vi "Test tools list.vi"(8 "error in (no error)":errorcluster) -> (0 "error out":errorcluster, 3 "body":string)   [LabVIEW 2020, in "MCP Server tests.lvlib"]
uses:
  MCP Server tests.lvlib
  <vilib>/JDP Science/JSONtext/Next JSON Value.vi
  <vilib>/JDP Science/JSONtext/String Subset.vi
  <vilib>/JDP Science/JSONtext/Parsing/Advance past next JSON Value (inlined COPY).vi
  <vilib>/JDP Science/JSONtext/Parsing/Advance past whitespace.vi
  <vilib>/JDP Science/JSONtext/Parsing/Advance past String.vi
  <vilib>/JDP Science/JSONtext/Parsing/Advance past Number.vi
  <vilib>/JDP Science/JSONtext/Parsing/Advance past Line Ending.vi
  <vilib>/JDP Science/JSONtext/Parsing/Parse Full Path or Item Name.vi
  <vilib>/JDP Science/JSONtext/Parsing/Advance past Array.vi
  <vilib>/JDP Science/JSONtext/Parsing/Advance past Object.vi
  <vilib>/JDP Science/JSONtext/support/Error Cluster From Code.vi
  <vilib>/JDP Science/JSONtext/Offset/Find Item Locations by Path.vi
  <vilib>/addons/_JKI Toolkits/Caraya/classes/Test/Test.lvclass
  <vilib>/addons/_JKI Toolkits/Caraya/classes/Assert/Assert.lvclass
  <vilib>/JDP Science/JSONtext/JSONtext.lvlib
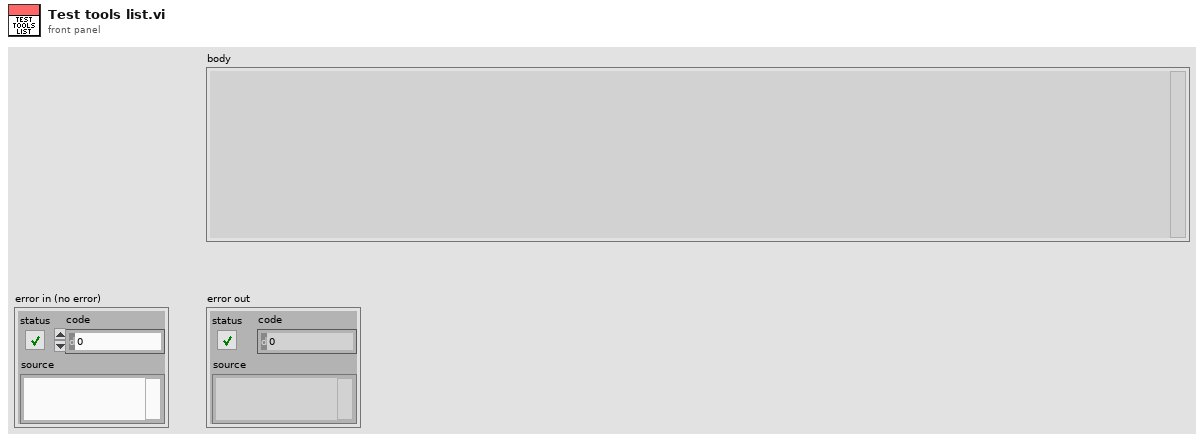
[diagram p1: front panel]
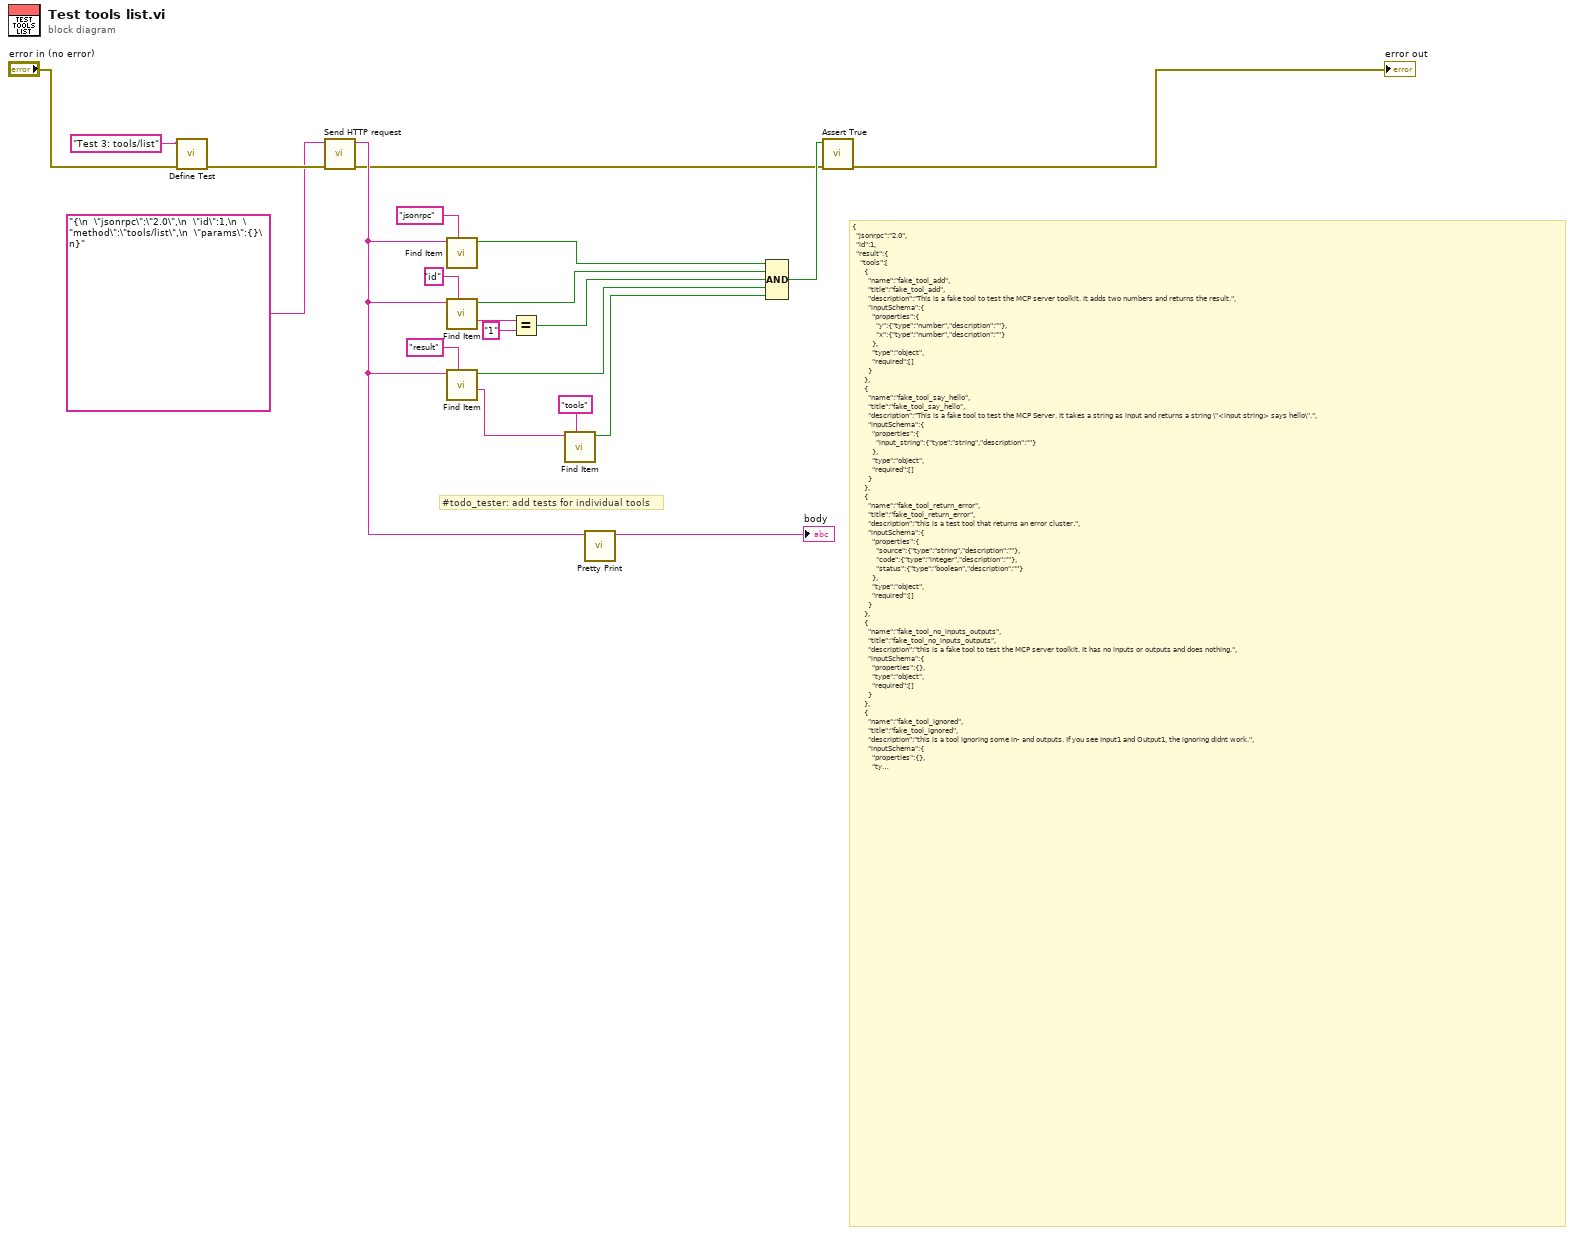
[diagram p0: block diagram]
diagram:
  # "#todo_tester: add tests for individual tools"
  # "{\n  \"jsonrpc\":\"2.0\",\n  \"id\":1,\n  \"result\":{\n    \"tools\":[\n      {\n        \"name\":\"fake_tool_add\",\n        \"title\":\"fake_tool_add\",\n        \"description\":\"This is a fake tool to test the MCP server toolkit. It adds two numbers and returns the result.\",\n        \"inputSchema\":{\n          \"properties\":{\n            \"y\":{\"type\":\"number\",\"description\":\"\"},\n            \"x\":{\"type\":\"number\",\"description\":\"\"}\n          },\n          \"type\":\"object\",\n          \"required\":[]\n        }\n      },\n      {\n        \"name\":\"fake_tool_say_hello\",\n        \"title\":\"fake_tool_say_hello\",\n        \"description\":\"This is a fake tool to test the MCP Server. It takes a string as input and returns a string \\\"<input string> says hello\\\".\",\n        \"inputSchema\":{\n          \"properties\":{\n            \"input_string\":{\"type\":\"string\",\"description\":\"\"}\n          },\n          \"type\":\"object\",\n          \"required\":[]\n        }\n      },\n      {\n        \"name\":\"fake_tool_return_error\",\n        \"title\":\"fake_tool_return_error\",\n        \"description\":\"this is a test tool that returns an error cluster.\",\n        \"inputSchema\":{\n          \"properties\":{\n            \"source\":{\"type\":\"string\",\"description\":\"\"},\n            \"code\":{\"type\":\"integer\",\"description\":\"\"},\n            \"status\":{\"type\":\"boolean\",\"description\":\"\"}\n          },\n          \"type\":\"object\",\n          \"required\":[]\n        }\n      },\n      {\n        \"name\":\"fake_tool_no_inputs_outputs\",\n        \"title\":\"fake_tool_no_inputs_outputs\",\n        \"description\":\"this is a fake tool to test the MCP server toolkit. It has no inputs or outputs and does nothing.\",\n        \"inputSchema\":{\n          \"properties\":{},\n          \"type\":\"object\",\n          \"required\":[]\n        }\n      },\n      {\n        \"name\":\"fake_tool_ignored\",\n        \"title\":\"fake_tool_ignored\",\n        \"description\":\"this is a tool ignoring some in- and outputs. If you see Input1 and Output1, the ignoring didnt work.\",\n        \"inputSchema\":{\n          \"properties\":{},\n          \"type\":\"object\",\n          \"required\":[]\n        }\n      }\n    ]\n  }\n}"
  n1 = call <vilib>:"Define Test.vi"("error in (no error)"="error in (no error)", "Label (VI Title)"="Test 3: tools/list") -> ("error out"=w8:errorcluster)  [unwired: 8 in, 1 out]
  n2 = call "Send HTTP request.vi"("error in (no error)"=w8, "request"="{\n  \"jsonrpc\":\"2.0\",\n  \"id\":1,\n  \"method\":\"tools/list\",\n  \"params\":{}\n}" ("buffer")) -> ("error out"=w9:errorcluster, "response"=w20:string)  [unwired: 7 in, 1 out]
  n3 = call <vilib>:"Find Item.vi"("$Path or Item Name"="jsonrpc", "JSON"=w20) -> ("Found"=w14:bool)  [unwired: 6 in, 3 out]
  n4 = call <vilib>:"Find Item.vi"("$Path or Item Name"="id", "JSON"=w20) -> ("<JSON>"=w12:string, "Found"=w15:bool)  [unwired: 6 in, 2 out]
  n5 = call <vilib>:"Find Item.vi"("$Path or Item Name"="result", "JSON"=w20) -> ("<JSON>"=w1:string, "Found"=w19:bool)  [unwired: 6 in, 2 out]
  n6 = Equal?(x=w12, y="1") -> (x = y?=w16:bool)
  n7 = call <vilib>:"Find Item.vi"("$Path or Item Name"="tools", "JSON"=w1) -> ("Found"=w2:bool)  [unwired: 6 in, 3 out]
  n8 = call <vilib>:"Pretty Print.vi"("JSON"=w20) -> ("<JSON>"=→"body":string)  [unwired: 8 in, 2 out]
  n9 = Compound Arithmetic op=AND(w14, w15, w16, w19, w2) -> (w17:bool)
  n10 = call <vilib>:"Assert True.vi"("error in (no error)"=w9, "True?"=w17) -> ("error out"=→"error out":errorcluster)  [unwired: 8 in, 1 out]
